vi "FormMain.vi"() -> ()   [LabVIEW 2012]
uses:
  S7Ref.vi
  resultShow.vi
panel:
  out "检具15":bool=TRUE
  out "取出工件":bool=TRUE
  out "判断是否合格":bool=TRUE
  out "检具15":bool=TRUE
  out "检具14":bool=TRUE
  out "检具13":bool=TRUE
  out "检具12":bool=TRUE
  out "扫码":bool
  in  "管柱码":string
  out "检具11":bool=TRUE
  in  "countLeft":u32
  out "检具7":bool
  out "检具8":bool=TRUE
  in  "判定设定 2":string[][](table)
  in  "参数设定 2":string[][](table)
  out "takesTime":string
  out "表格控件":string[][](table)
  out "FFT范围 2":string[][](table)
  out "压力损失":bool
  out "外泄漏":bool
  out "检具9":bool
  out "检具10":bool=TRUE
  out "检具2":bool
  out "输出扭矩":dbl caption="数值 24" format="%.1f Nm"
  in  "打开按钮":bool
  in  "自动":bool
  out "rigStatus":string="提示信息"
  out "connectionMode":string
  out "productsName":string
  out "userStatus":string
  out "userName":string
  out "放入工件":bool
  out "检具1":bool=TRUE
  out "检具3":bool
  out "检具4":bool
  out "检具5":bool
  out "检具6":bool
  # "广东和氏自动化技术股份有限公司"
  # "总成检验专机"
  # "GUANGDONG HESH AUTOMATION TECHNOLOGY CO.,LTD."
  # "步骤"
  # "完成计数："
  # "用时："
  # "："
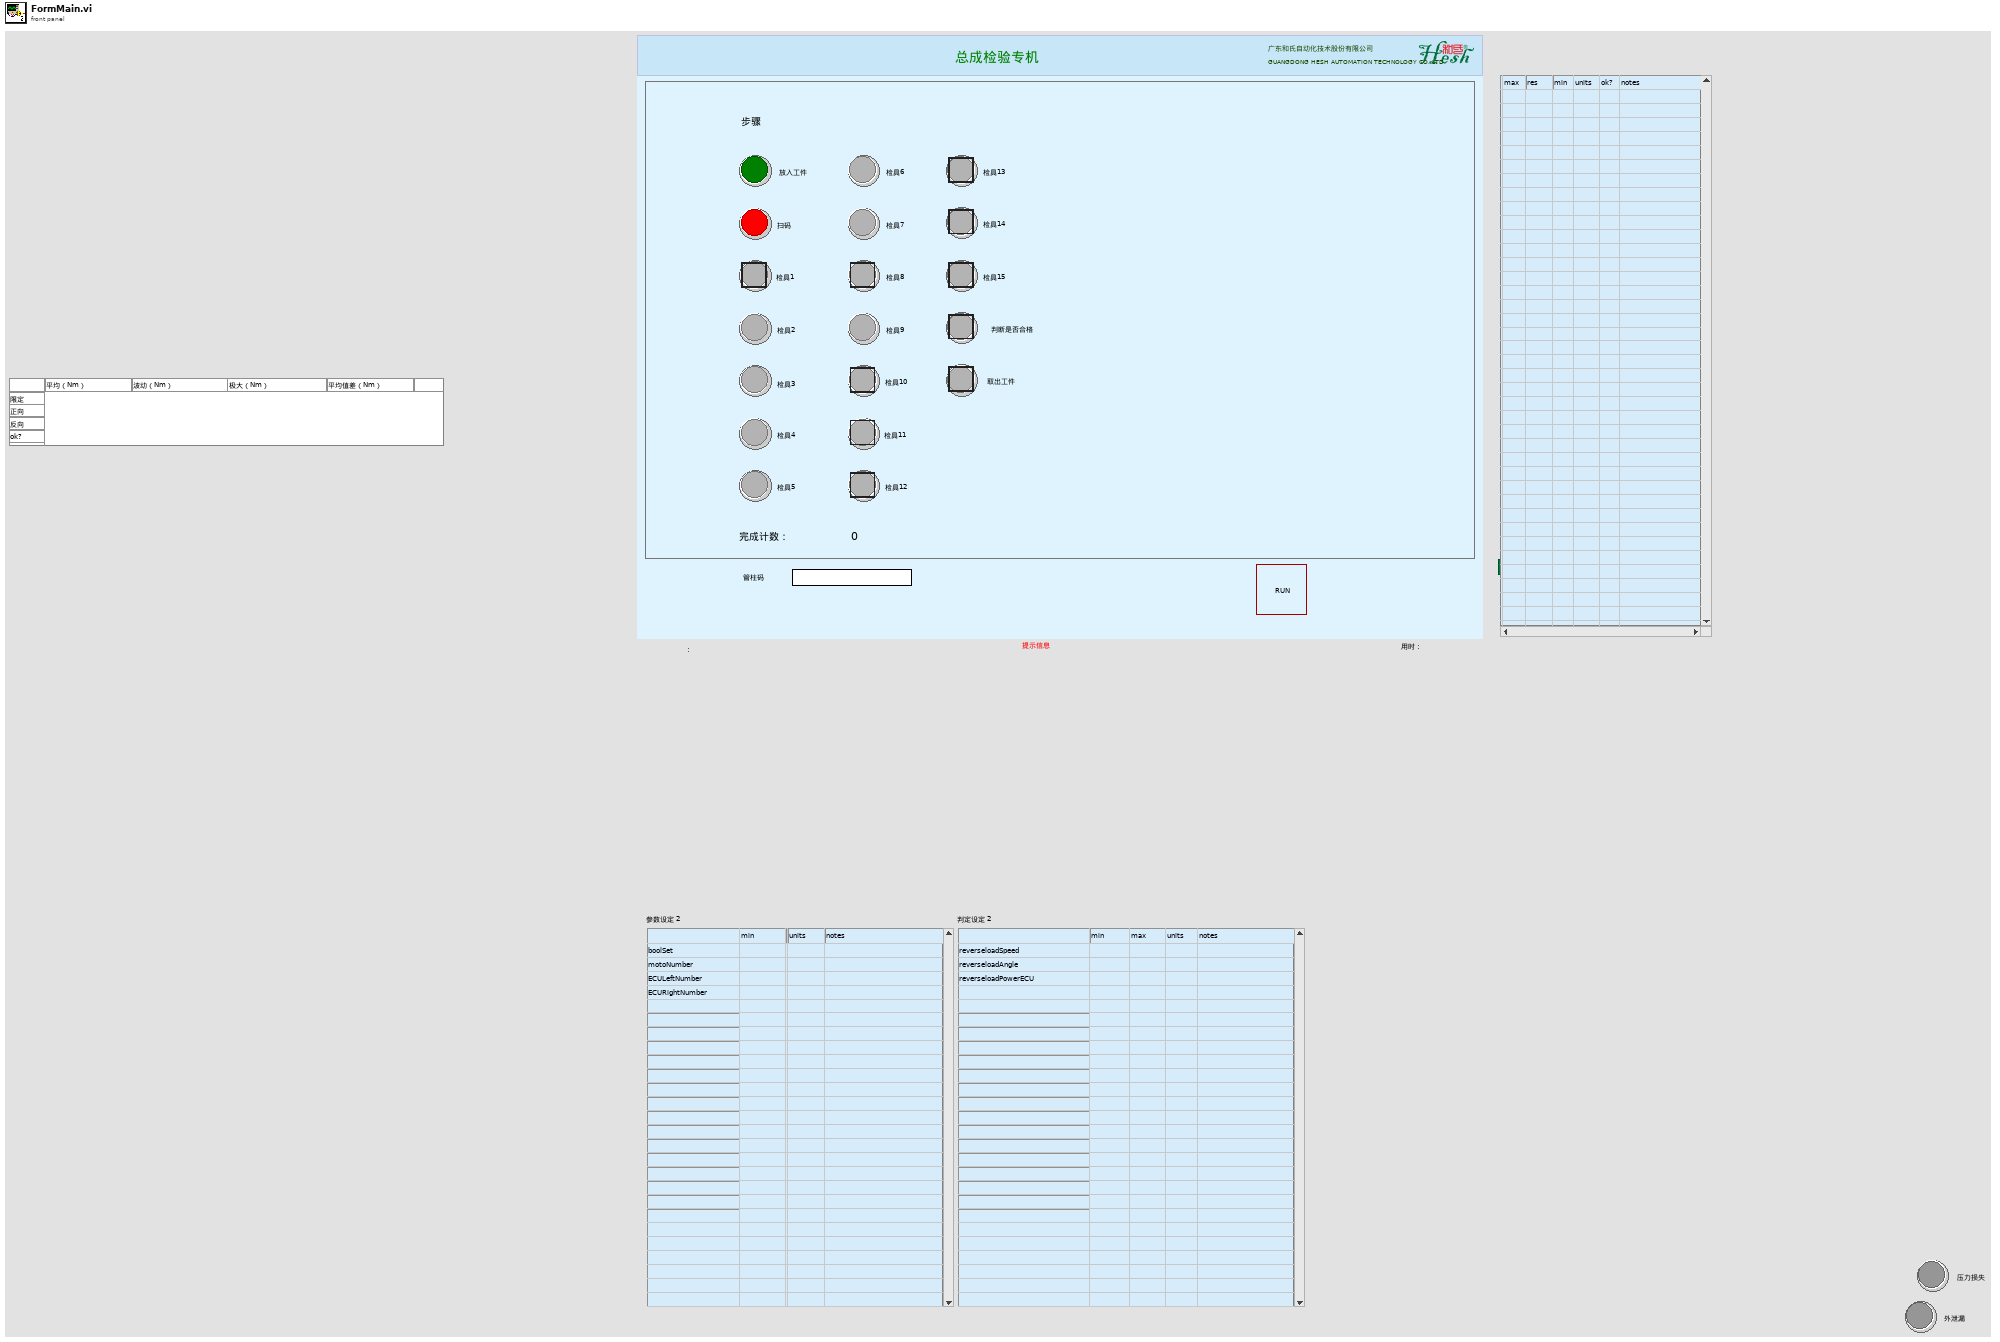
[diagram p1: front panel]
types:
  T1 = enum32{"Invalid", "Standard", "Closed", "Hidden", "Minimized", "Maximized"}
  T2 = cluster{"takesTime":refnum<vi>, "userStatus":refnum<vi>, "userName":refnum<vi>, "connectionMode":refnum<vi>, "productsName":refnum<vi>, "rigStatus":refnum<vi>, "管柱码":refnum<vi>}
  T3 = cluster{"userCode":string, "userName":string, "userStatus":string, "connectionMode":string, "takesTime":string, "countDone":string, "countOK":string, "countNG":string, "rigStatus":string, "productsName":string, "partCode1":string, "partCode2":string, "partCode3":string}
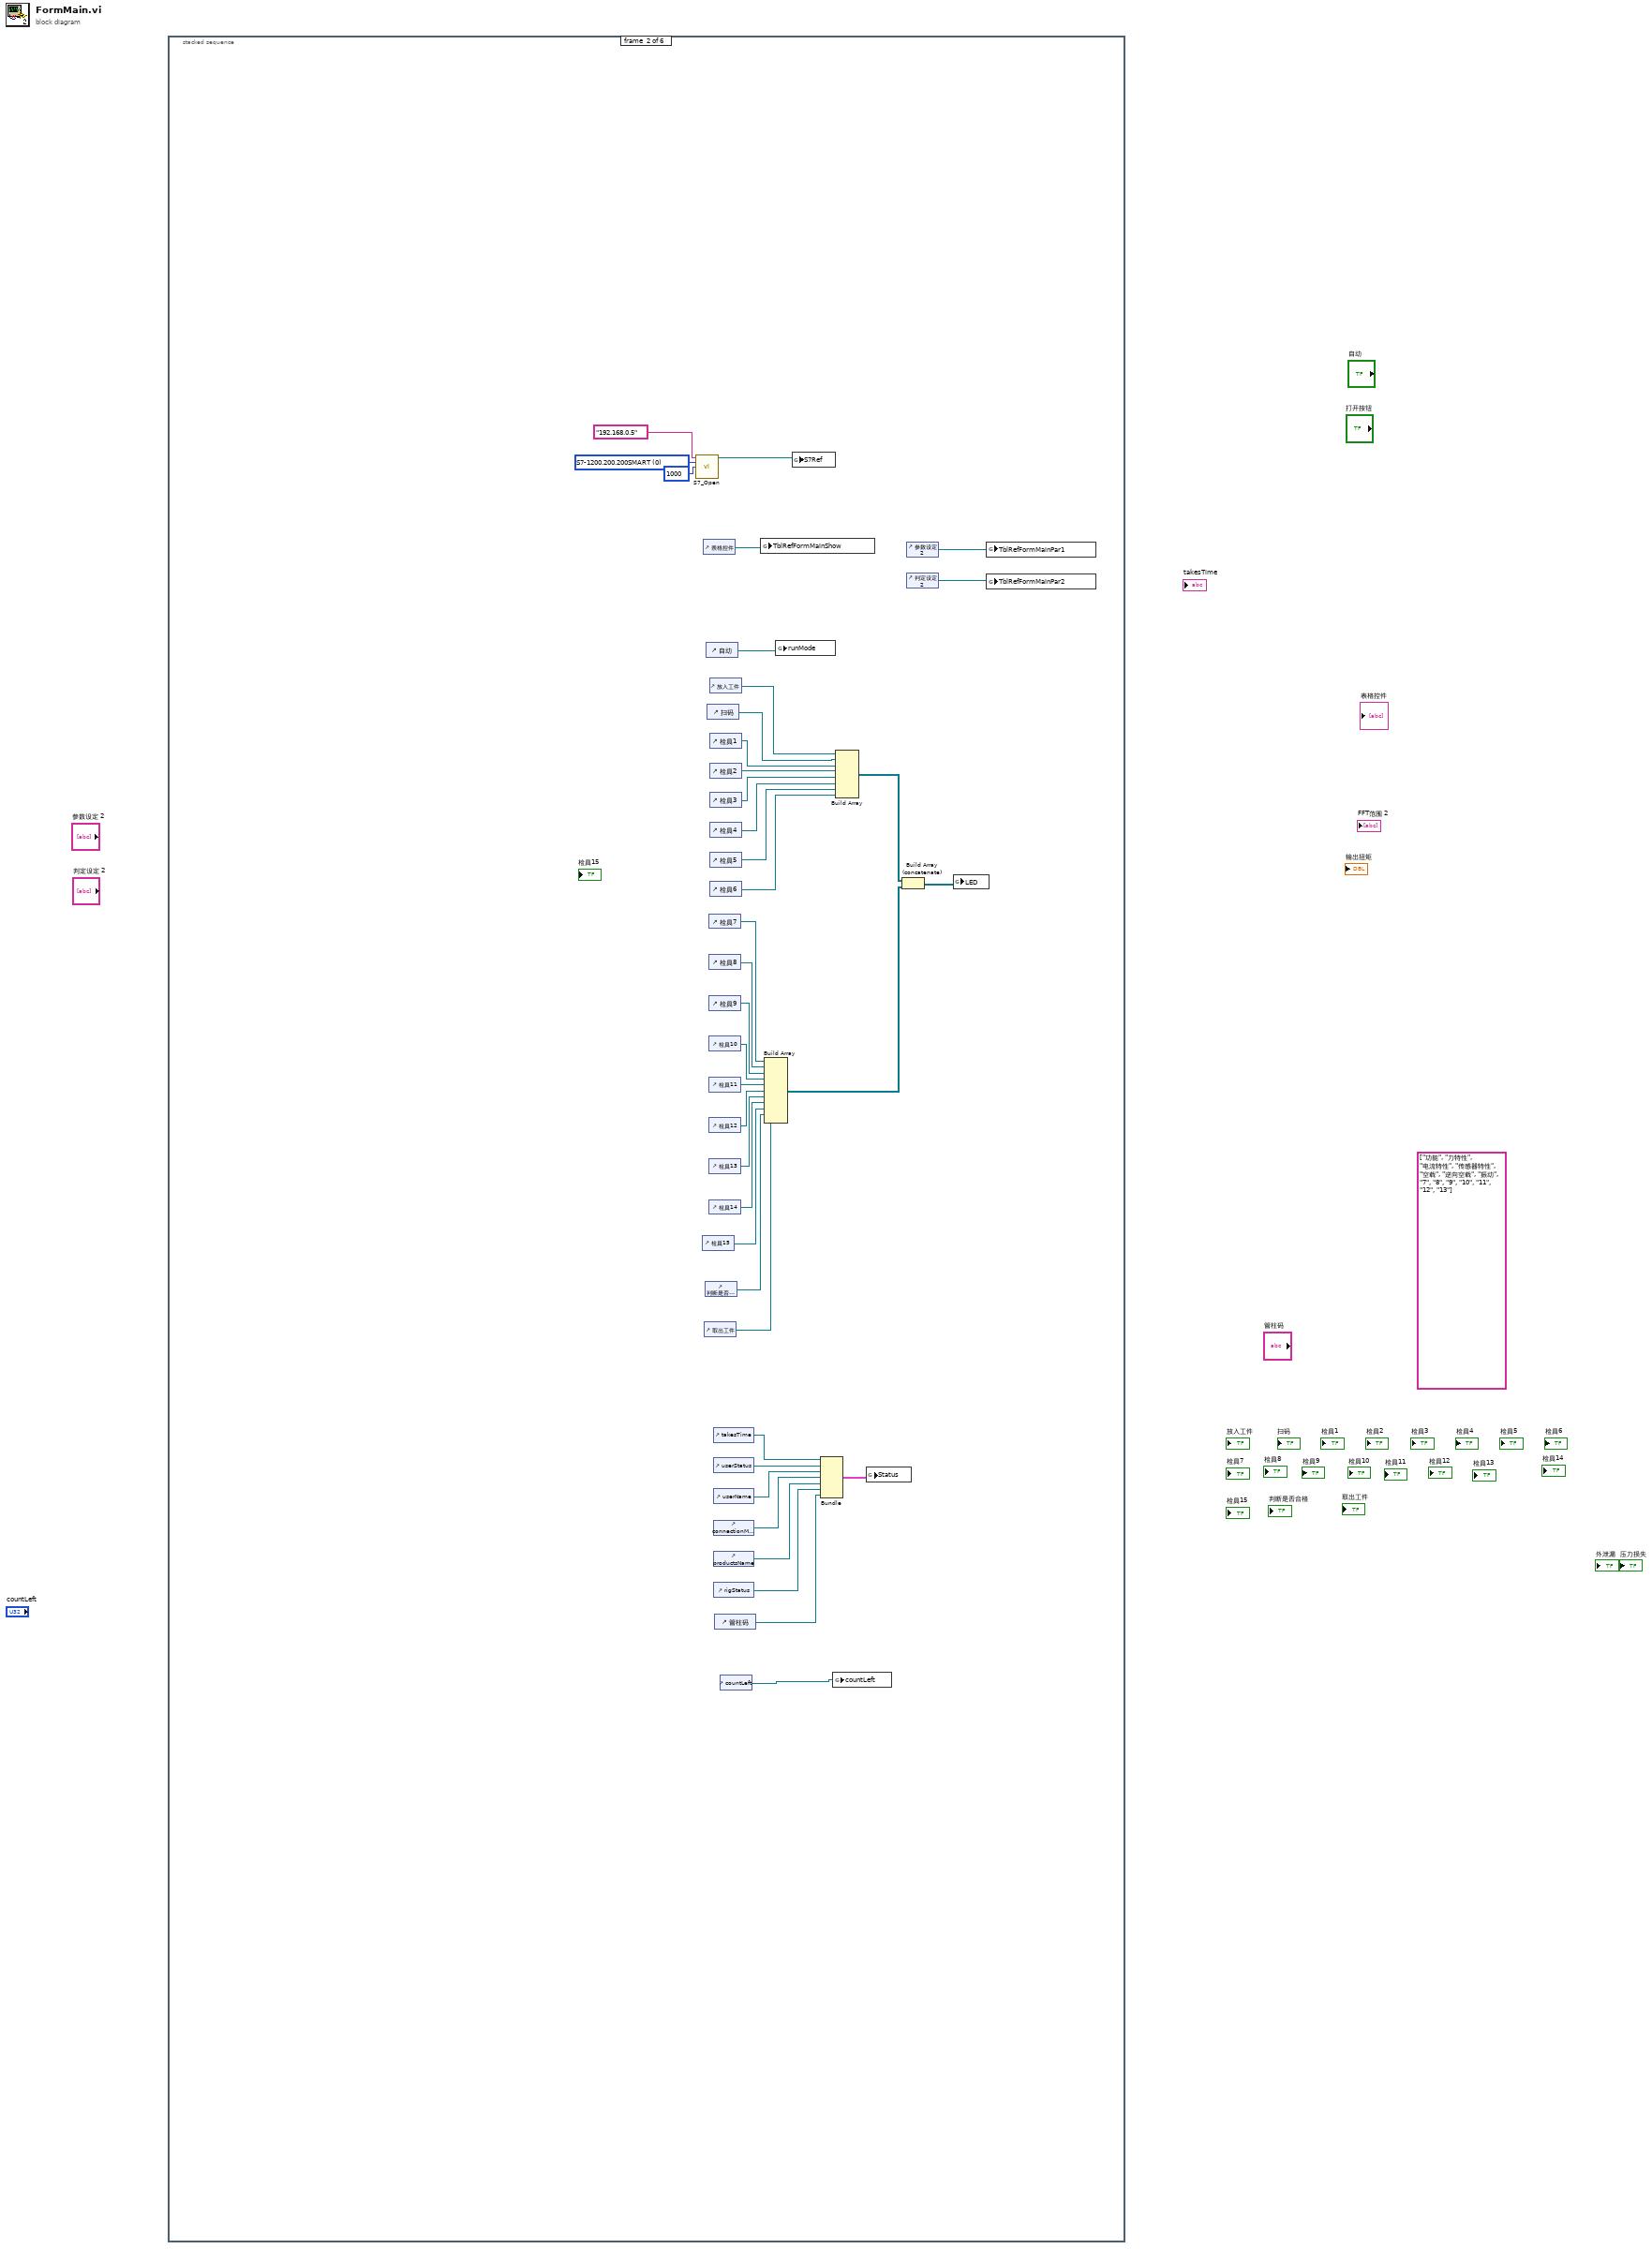
[diagram p0: block diagram]
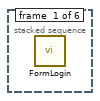
[diagram p2: hidden frame]
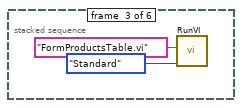
[diagram p3: hidden frame]
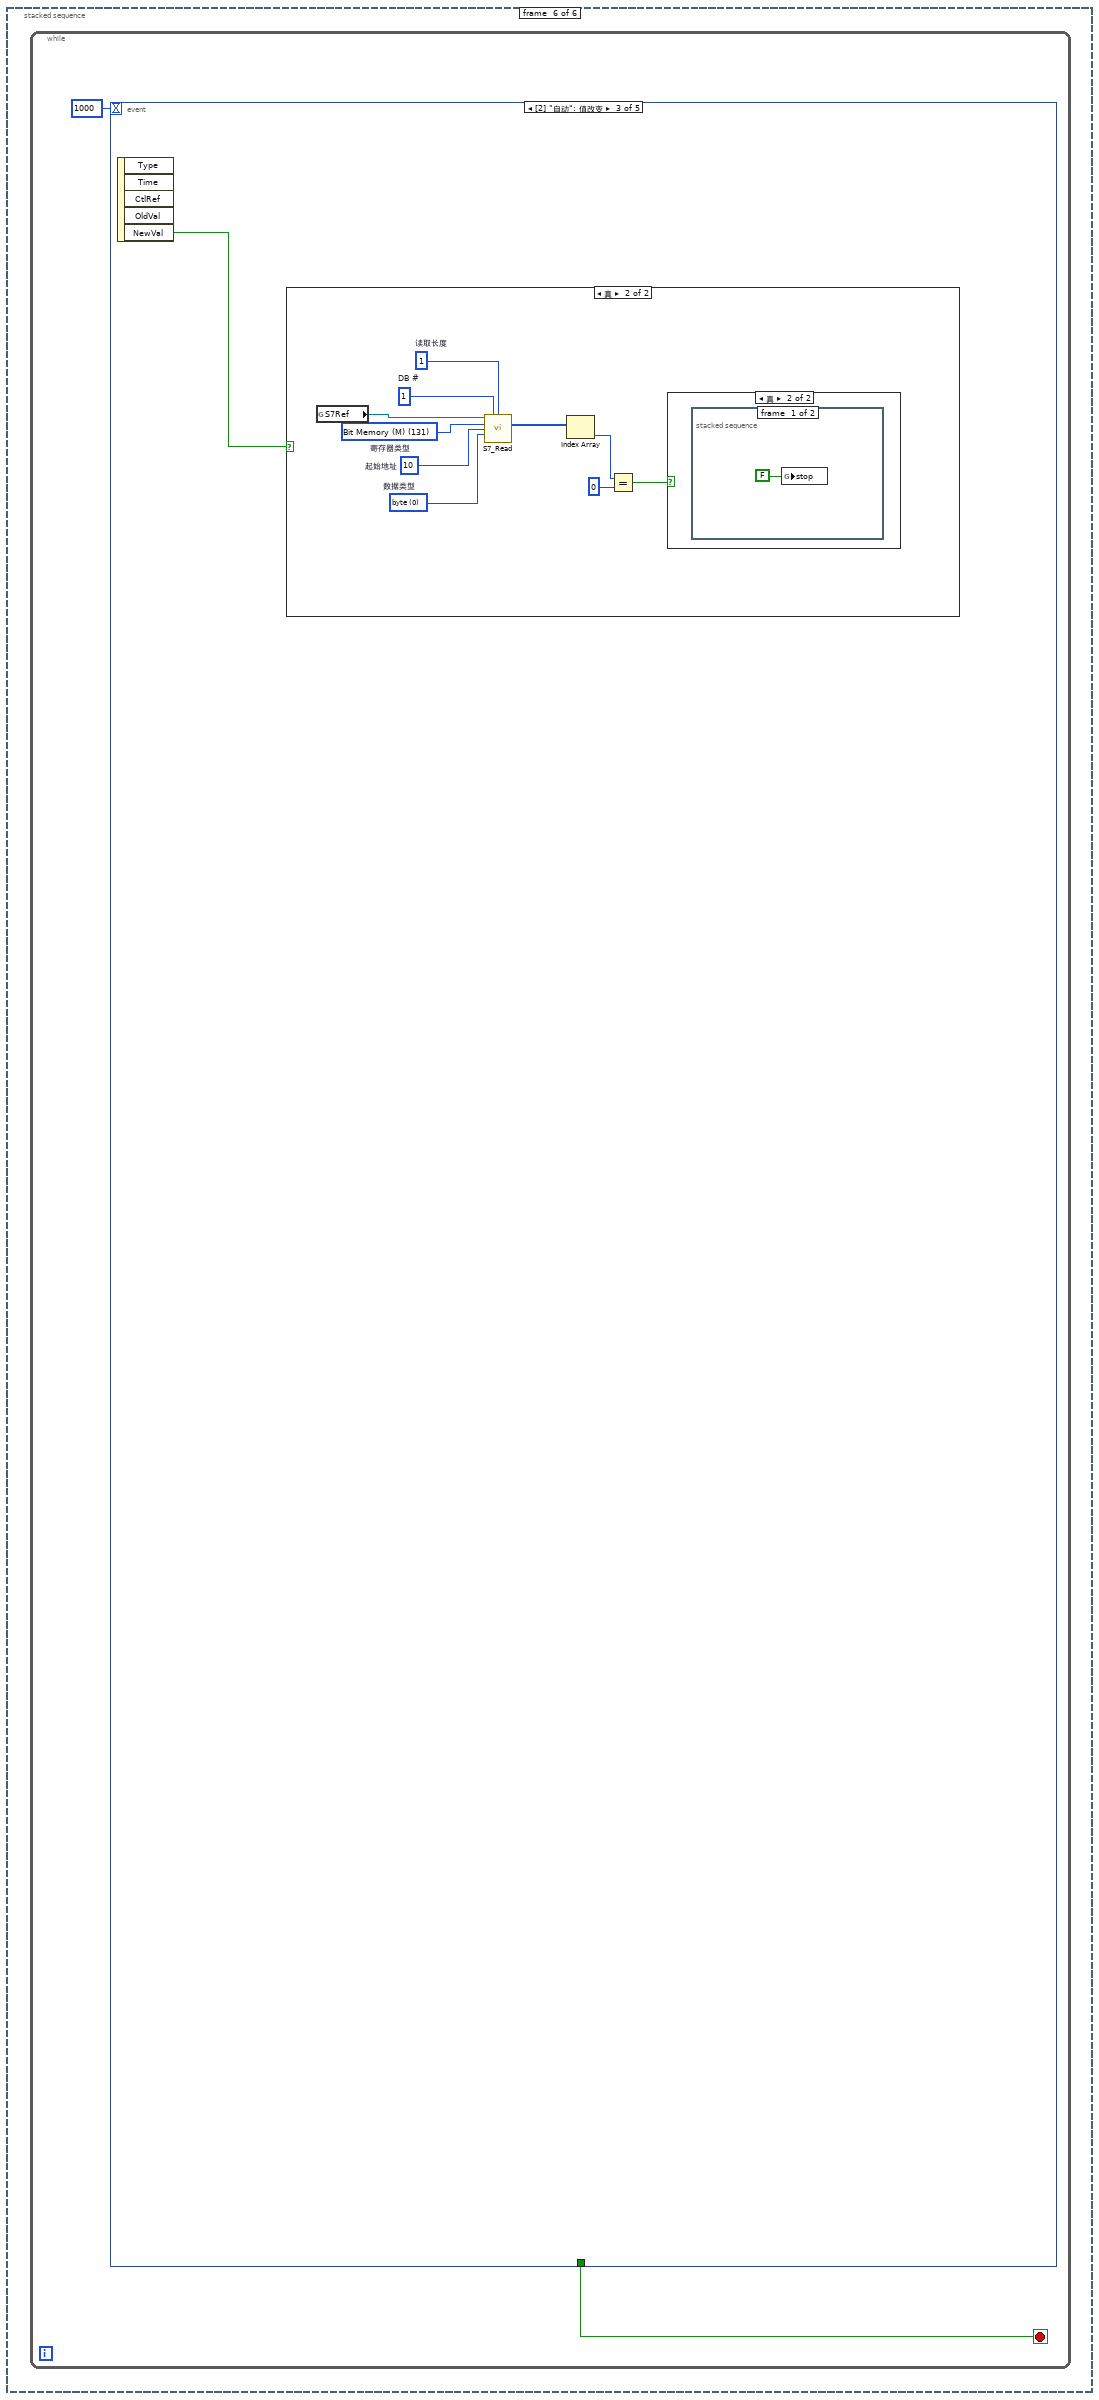
[diagram p6: hidden frame]
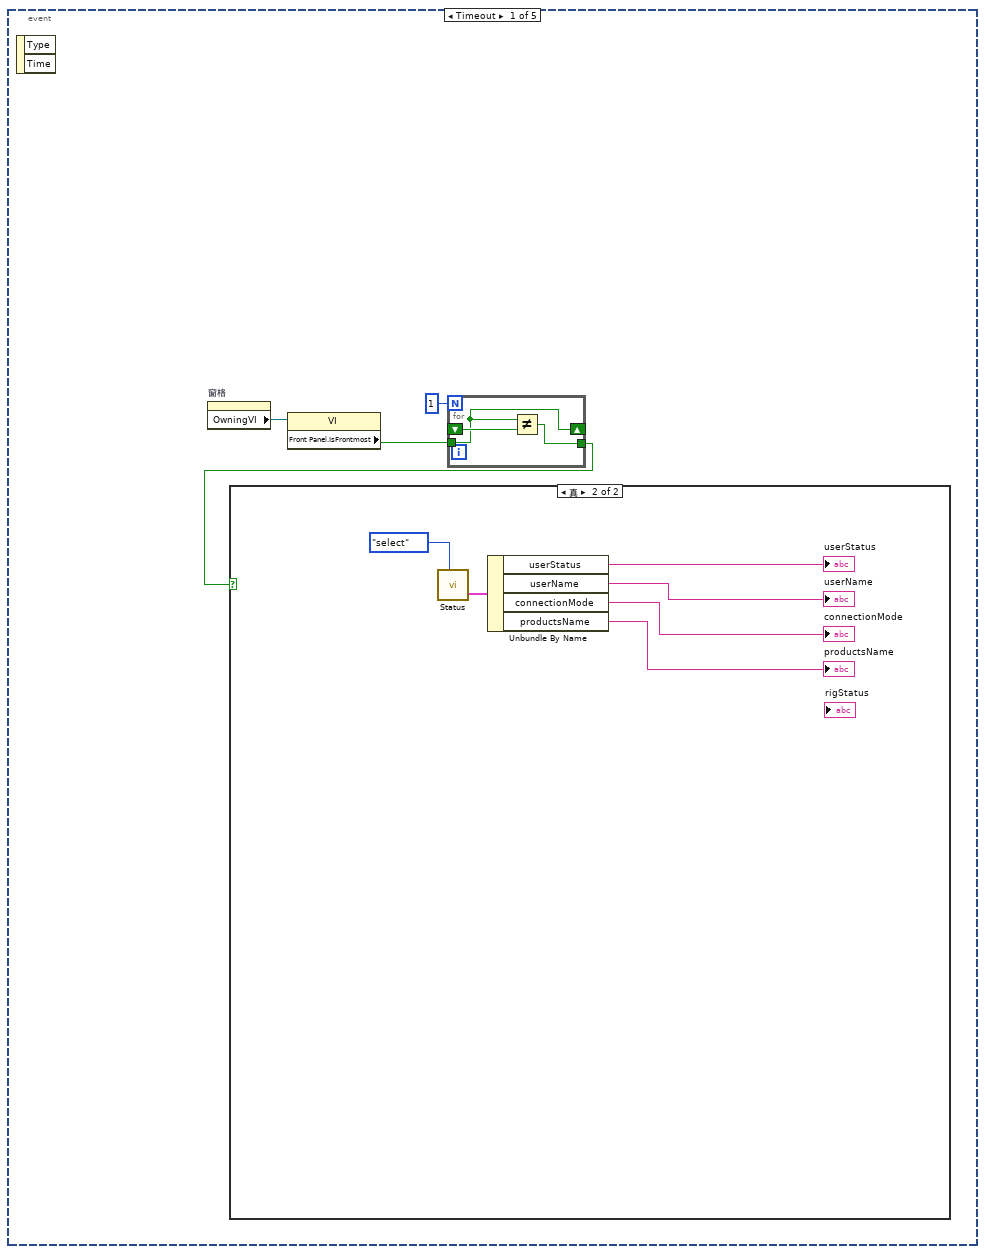
[diagram p7: hidden frame]
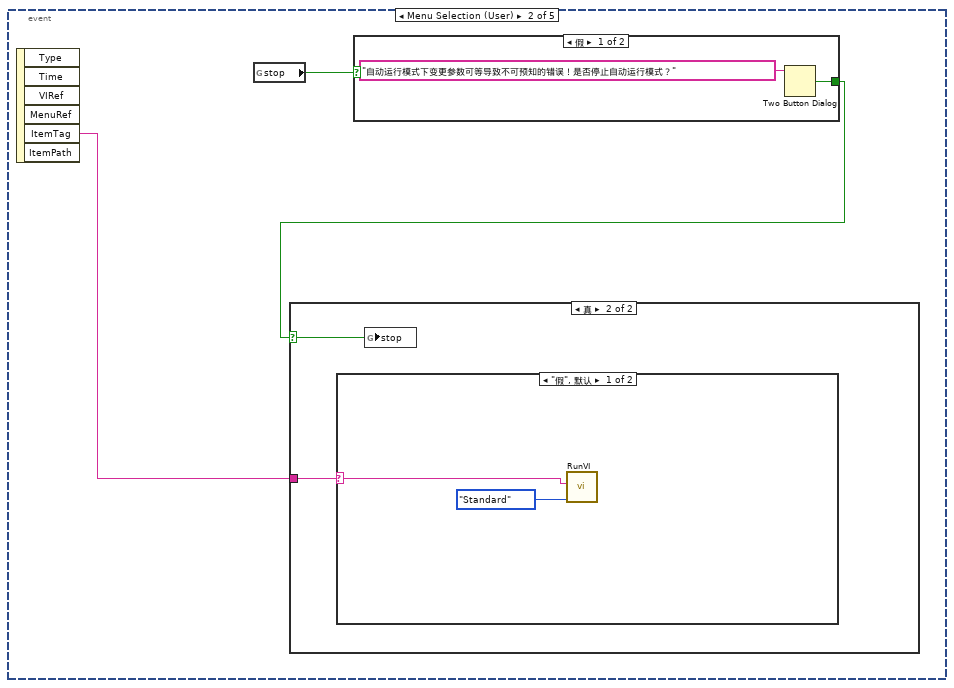
[diagram p9: hidden frame]
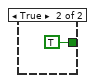
[diagram p10: hidden frame]
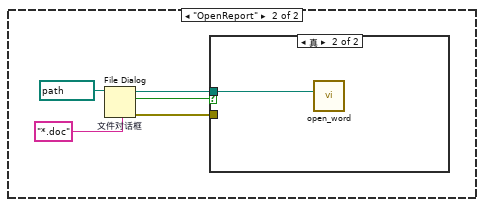
[diagram p12: hidden frame]
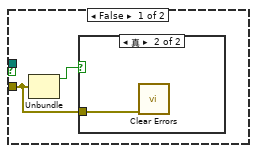
[diagram p13: hidden frame]
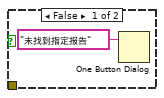
[diagram p14: hidden frame]
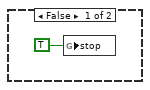
[diagram p15: hidden frame]
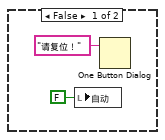
[diagram p16: hidden frame]
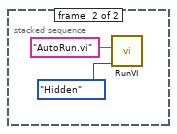
[diagram p17: hidden frame]
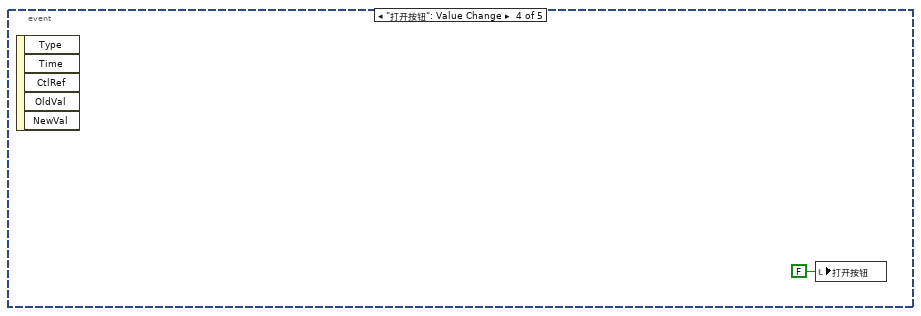
[diagram p18: hidden frame]
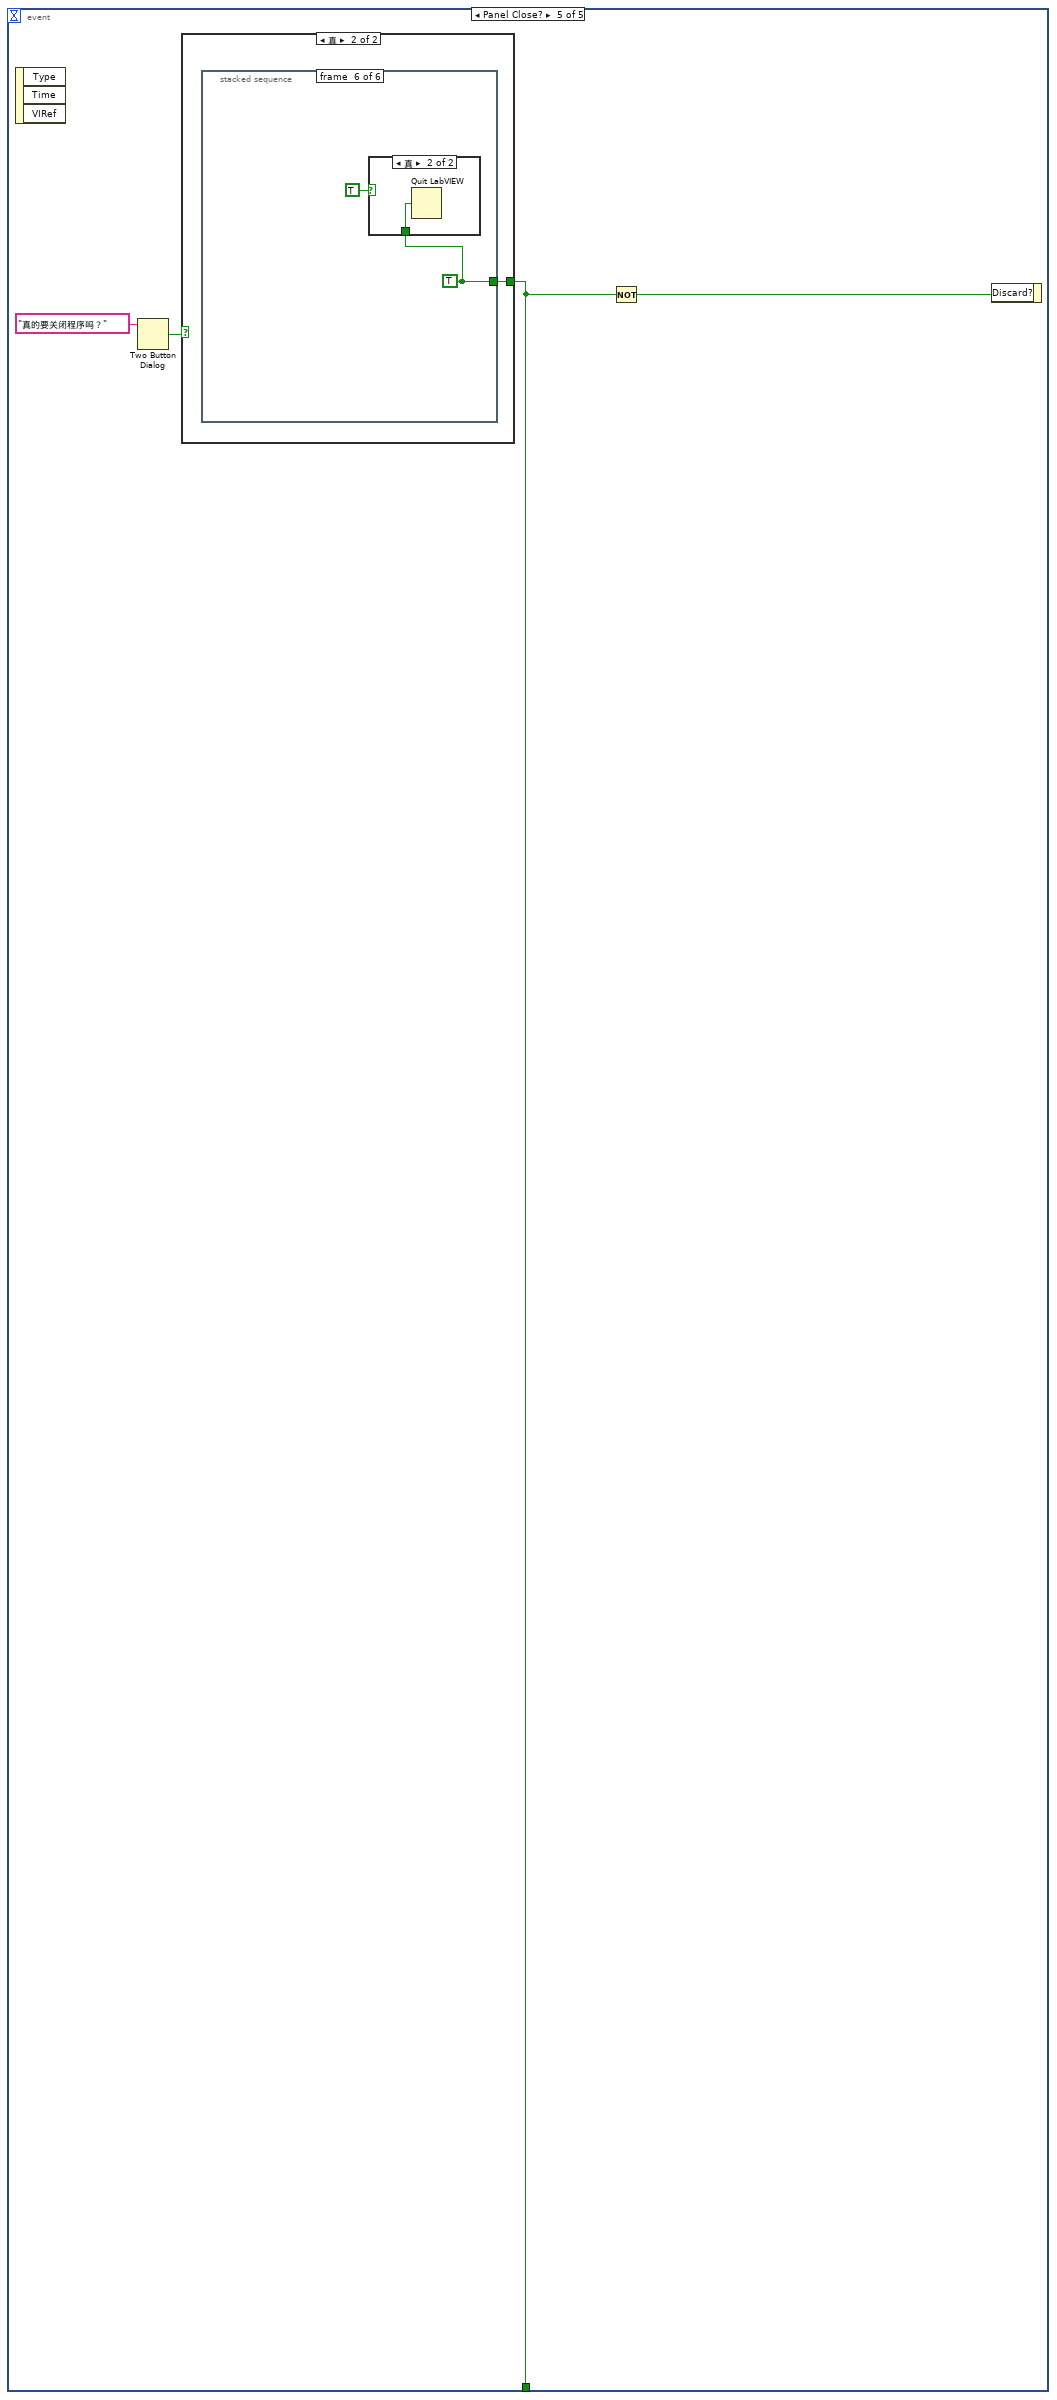
[diagram p19: hidden frame]
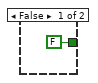
[diagram p20: hidden frame]
diagram:
  (unwired) string[] ["功能", "力特性", "电流特性", "传感器特性", "空载", "逆向空载", "振动", "7", "8", "9", "10", "11", "12", "13"] ("字符串[]")
  n1 = stacked-sequence {
    frame #0 {
      n2 = call "FormLogin.vi"() -> ()  [unwired: 12 in]
    }
    frame #1 {
      w37 = u8 0 items=["S7-1200.200.200SMART"=0, "S7-300"=2, "S7-400"=3] ("PLC 系列")
      n3 = call "S7_Open.vi"("IP 地址"="192.168.0.5", "PLC 系列"=w37, "超时（MS）"=1000) -> ("TCP"=w35:refnum<k5>)  [unwired: 10 in, 2 out]
      n4 = control-ref of="检具15"() -> (w3:refnum<vi>)
      n5 = control-ref of="表格控件"() -> (w39:refnum<vi>)
      n6 = control-ref of="取出工件"() -> (w1:refnum<vi>)
      n7 = control-ref of="判断是否合格"() -> (w2:refnum<vi>)
      n8 = control-ref of="自动"() -> (w34:refnum<vi>)
      n9 = control-ref of="扫码"() -> (w10:refnum<vi>)
      n10 = control-ref of="检具7"() -> (w15:refnum<vi>)
      n11 = control-ref of="检具8"() -> (w14:refnum<vi>)
      n12 = control-ref of="检具9"() -> (w9:refnum<vi>)
      n13 = control-ref of="检具10"() -> (w8:refnum<vi>)
      n14 = control-ref of="检具11"() -> (w7:refnum<vi>)
      n15 = control-ref of="检具12"() -> (w6:refnum<vi>)
      n16 = control-ref of="检具13"() -> (w4:refnum<vi>)
      n17 = control-ref of="检具14"() -> (w5:refnum<vi>)
      n18 = control-ref of="放入工件"() -> (w11:refnum<vi>)
      n19 = control-ref of="检具1"() -> (w28:refnum<vi>)
      n20 = control-ref of="检具2"() -> (w29:refnum<vi>)
      n21 = control-ref of="检具3"() -> (w30:refnum<vi>)
      n22 = control-ref of="检具4"() -> (w31:refnum<vi>)
      n23 = control-ref of="检具5"() -> (w32:refnum<vi>)
      n24 = control-ref of="检具6"() -> (w33:refnum<vi>)
      n25 = control-ref of="takesTime"() -> (w21:refnum<vi>)
      n26 = control-ref of="userStatus"() -> (w27:refnum<vi>)
      n27 = control-ref of="userName"() -> (w26:refnum<vi>)
      n28 = control-ref of="connectionMode"() -> (w25:refnum<vi>)
      n29 = control-ref of="productsName"() -> (w24:refnum<vi>)
      n30 = control-ref of="rigStatus"() -> (w23:refnum<vi>)
      n31 = control-ref of="管柱码"() -> (w12:refnum<vi>)
      n32 = control-ref of="countLeft"() -> (w13:refnum<vi>)
      n33 = global write "resultShow.vi" "TblRefFormMainShow"(w39) -> ()
      n34 = Build Array(w15, w14, w9, w8, w7, w6, w4, w5, w3, w2, w1) -> (w16:refnum<vi>[])
      n35 = global write "resultShow.vi" "runMode"(w34) -> ()
      n36 = global write "S7Ref.vi" "S7Ref"(w35) -> ()
      n37 = Bundle("takesTime"=w21, "userStatus"=w27, "userName"=w26, "connectionMode"=w25, "productsName"=w24, "rigStatus"=w23, "管柱码"=w12) -> (w22:T2)  [unwired: 1 in]
      n38 = global write "resultShow.vi" "countLeft"(w13) -> ()
      n39 = Build Array(w11, w10, w28, w29, w30, w31, w32, w33) -> (w17:refnum<vi>[])
      n40 = global write "resultShow.vi" "Status"(w22) -> ()
      n41 = Build Array (concatenate)(w17, w16) -> (w18:refnum<vi>[])
      n42 = control-ref of="参数设定 2"() -> (w20:refnum<vi>)
      n43 = control-ref of="判定设定 2"() -> (w19:refnum<vi>)
      n44 = global write "resultShow.vi" "LED"(w18) -> ()
      n45 = global write "resultShow.vi" "TblRefFormMainPar1"(w20) -> ()
      n46 = global write "resultShow.vi" "TblRefFormMainPar2"(w19) -> ()
    }
    frame #2 {
      n47 = call "RunVI.vi"("状态"=T1."Standard", "名称或相对路径"="FormProductsTable.vi") -> ()  [unwired: 9 in, 1 out]
    }
    frame #3 {
    }
    frame #4 {
    }
    frame #5 {
      n48 = while {
        stop <- w43 stop-if-true
        n49 = event shown="[2] \"自动\": 值改变" {
          selector: _ -> [_ _ _ _ _]
          dyn-events: _ -> [_ _ _ _ _]
          timeout: 1000 -> [_ _ _ _ _]
          tunnel: [_ _ _ _ w95] -> w43
          event Timeout {
            n50 = event-data() -> ()  [unwired: 1 in, 2 out]
            n51 = property on="窗格" class="Pane"() -> ("OwningVI"=w47:refnum<vi>)  [unwired: 2 in, 2 out]
            n52 = property class="VI"(reference=w47) -> ("Front Panel.IsFrontmost"=w45:bool)  [unwired: 1 in, 2 out]
            n53 = for {
              N: 1 -> [_]
              shift-right: [w55] -> _
              shift-left: _ -> [w56]
              tunnel: w45 -> [w55]
              tunnel: [w54] -> w44
              n54 = Not Equal?(x=w55, y=w56) -> (x != y?=w54:bool)
            }
            n55 = case shown="真" w44 {
              frame False {
              }
              frame True {
                n56 = call "Status.vi"("模式"=enum16{"select", "insert", "update", "delete"}."select") -> ("元素"=w52:T3)  [unwired: 10 in]
                n57 = Unbundle By Name(w52) -> ("userStatus"=→"userStatus":string, "userName"=→"userName":string, "connectionMode"=→"connectionMode":string, "productsName"=→"productsName":string)
              }
            }
          }
          event Menu Selection (User) {
            n58 = event-data() -> ("ItemTag"=w59:string)  [unwired: 1 in, 5 out]
            n59 = global read "全局 3.vi" "stop"() -> (w58:bool)
            n60 = case shown="假" w58 {
              tunnel: [w60 TRUE ("T button?")] -> w57
              frame False {
                n61 = Two Button Dialog(message="自动运行模式下变更参数可等导致不可预知的错误！是否停止自动运行模式？" ("消息")) -> (T button?=w60:bool)  [unwired: 2 in]
              }
              frame True {
              }
            }
            n62 = case shown="真" w57 {
              selector: w57 -> [_ w63]
              tunnel: w59 -> [_ w64]
              frame False {
              }
              frame True {
                n63 = case shown="\"假\", 默认" w64 {
                  selector: w64 -> [w65 _]
                  frame "假", Default {
                    n64 = call "RunVI.vi"("状态"=T1."Standard", "名称或相对路径"=w65) -> ()  [unwired: 9 in, 1 out]
                  }
                  frame "OpenReport" {
                    n65 = File Dialog "文件对话框"(6:"*.doc" ("prompt"), 11:path "D:/报表" ("开始路径")) -> (0:w67:errorcluster, 2:w69:bool, 3:w68:path)  [unwired: 1 in, 5 out]
                    n66 = case shown="真" w69 {
                      tunnel: w68 -> [_ w76]
                      tunnel: w67 -> [w72 _]
                      frame False {
                        n67 = Unbundle(w72) -> ("status"=w73:bool)  [unwired: 2 out]
                        n68 = case shown="真" w73 {
                          tunnel: w72 -> [_ w75]
                          frame False {
                            n69 = One Button Dialog(message="未找到指定报告" ("消息")) -> ()  [unwired: 1 in, 1 out]
                          }
                          frame True {
                            n70 = call <vilib>:"Clear Errors.vi"("error in (no error)"=w75) -> ()  [unwired: 6 in, 1 out]
                          }
                        }
                      }
                      frame True {
                        n71 = call "open_word.vi"("所选路径"=w76) -> ()  [unwired: 11 in]
                      }
                    }
                  }
                }
                n72 = global write "全局 3.vi" "stop"(w63) -> ()
              }
            }
          }
          event "自动": Value Change {
            n73 = event-data() -> ("NewVal"=w77:bool)  [unwired: 1 in, 4 out]
            n74 = case shown="真" w77 {
              frame False {
                n75 = global write "全局 3.vi" "stop"(TRUE ("布尔 1")) -> ()
              }
              frame True {
                w82 = u32 10  # 起始地址
                w84 = u16 0 items=["byte", "word", "Dword"]  # 数据类型
                w85 = u8 131 items=["I/O (P)"=128, "Input (I)"=129, "Output (Q)"=130, "Bit Memory (M)"=131, "Data (DB)"=132, "Instance Data (DI)"=133, "Local Data (L)"=134, "Predecessor Local Data (VL)"=135]  # 寄存器类型
                w86 = u16 1  # 读取长度
                w87 = u16 1  # DB #
                n76 = global read "S7Ref.vi" "S7Ref"() -> (w88:refnum<k5>)
                n77 = call "S7_Read.vi"("TCP"=w88, "DB #"=w87, "读取长度"=w86, "寄存器类型"=w85, "起始地址"=w82, "数据类型"=w84) -> ("数据"=w83:u32[])  [unwired: 6 in, 3 out]
                n78 = Index Array(array=w83) -> (element=w81:u32)  [unwired: 1 in]
                n79 = Equal?(x=w81, y=u32 0) -> (x = y?=w79:bool)
                n80 = case shown="真" w79 {
                  frame False {
                    n81 = local write "自动"(FALSE ("自动")) -> ()
                    n82 = One Button Dialog(message="请复位！" ("消息")) -> ()  [unwired: 1 in, 1 out]
                  }
                  frame True {
                    n83 = stacked-sequence {
                      frame #0 {
                        n84 = global write "全局 3.vi" "stop"(FALSE ("布尔 1")) -> ()
                      }
                      frame #1 {
                        n85 = call "RunVI.vi"("状态"=T1."Hidden", "名称或相对路径"="AutoRun.vi") -> ()  [unwired: 9 in, 1 out]
                      }
                    }
                  }
                }
              }
            }
          }
          event "打开按钮": Value Change {
            n86 = event-data() -> ()  [unwired: 1 in, 5 out]
            n87 = local write "打开按钮"(FALSE ("打开按钮")) -> ()
          }
          event Panel Close? {
            n88 = event-data() -> ()  [unwired: 1 in, 3 out]
            n89 = Two Button Dialog(message="真的要关闭程序吗？" ("消息")) -> (T button?=w96:bool)  [unwired: 2 in]
            n90 = case shown="真" w96 {
              tunnel: [FALSE w100] -> w95
              frame False {
              }
              frame True {
                n91 = stacked-sequence {
                  tunnel: [_ _ _ _ _ w108] -> w100
                  frame #0 {
                    n92 = for {
                      tunnel: string[] ["AutoRun.vi", "FormCamera.vi"] -> [w102] mode=indexing
                      n93 = call "CloseVI.vi"("名称或相对路径"=w102) -> ()  [unwired: 10 in, 1 out]
                    }
                  }
                  frame #1 {
                    n94 = shared-variable ".\\共享变量.lvlib\\string_5"("关闭程序中" ("string_5")) -> ()  [unwired: 1 in, 1 out]
                    n95 = global write "全局 3.vi" "stop"(TRUE ("布尔 2")) -> ()
                  }
                  frame #2 {
                    n96 = Wait (ms)(milliseconds to wait=u32 500 ("等待时间（毫秒）")) -> ()  [unwired: 1 out]
                  }
                  frame #3 {
                  }
                  frame #4 {
                    n97 = global read "S7Ref.vi" "S7Ref"() -> (w106:refnum<k5>)
                    n98 = call "S7_Close.vi"("TCP Connection Ref"=w106) -> ()  [unwired: 10 in, 1 out]
                  }
                  frame #5 {
                    w108 = TRUE
                    n99 = case shown="真" TRUE {
                      tunnel: w108 -> [_ w109]
                      frame False {
                      }
                      frame True {
                        n100 = Quit LabVIEW(quit? (T)=w109) -> ()
                      }
                    }
                  }
                }
              }
            }
            n101 = Not(x=w95) -> (.not. x?=w97:bool)
            n102 = event-data("Discard?"=w97) -> ()  [unwired: 1 in, 1 out]
          }
        }
      }
    }
  }
